vi "FTS Get Instrument Property Available Gain Levels.vi"(8 "error in (no error)":errorcluster, 10 "GainLevels":dbl[](array[numeric]), 11 "specIndex":u16) -> (0 "error out":errorcluster, 2 "GainLevels out":dbl[](array[numeric]), 3 "function return":u32)   [LabVIEW 2010, in "FTSLib.lvlib"]
doc: "unsigned int __cdecl FTS_GetInstrumentProperty_AvailableGainLevels(unsigned short specIndex, double* GainLevels);"
uses:
  FTSLib.lvlib
  FTSLib.dll
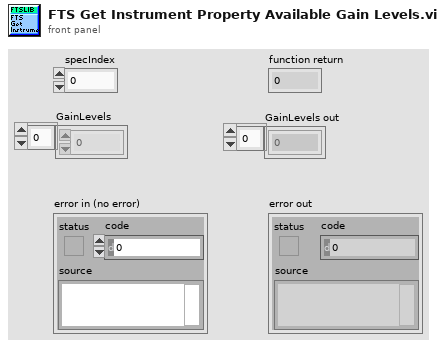
[diagram p1: front panel]
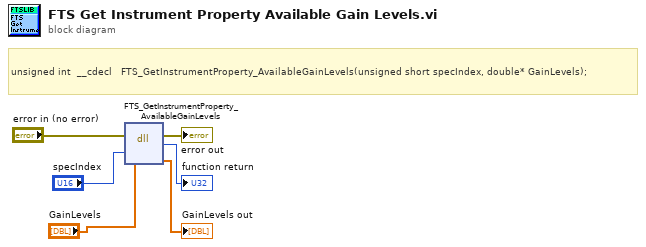
[diagram p0: block diagram]
diagram:
  # "unsigned int\t\t__cdecl   FTS_GetInstrumentProperty_AvailableGainLevels(unsigned short specIndex, double* GainLevels);"
  n1 = dll-call lib="FTSLib.*" fn="FTS_GetInstrumentProperty_AvailableGainLevels"(error in="error in (no error)", "specIndex"="specIndex", "GainLevels"="GainLevels") -> (error out=→"error out":errorcluster, "return type"=→"function return":u32, "GainLevels"=→"GainLevels out":dbl[])  [unwired: 3 in, 1 out]
